vi "Create Hardware Configuration.vi"   [LabVIEW 2018]
uses:
  Resources/Type Defs/Stage Configuration.ctl
  Resources/Type Defs/Microscope Configuration.ctl
  Resources/Type Defs/Microscope Type.ctl
  Resources/Type Defs/Virtual Camera Configuration.ctl
  Resources/Type Defs/Camera Type.ctl
  Resources/Type Defs/Laser Configuration.ctl
  Resources/Type Defs/Pump Configuration.ctl
  Resources/Type Defs/Hardware Configuration.ctl
  Resources/Type Defs/Shutter Configuration.ctl
  Resources/Type Defs/Physical Camera Assignment.ctl
  <vilib>/Utility/xml.llb/Write to XML File(string).vi
panel:
  # "Open the Block Diagram (Ctrl-E)\nto edit configuration settings."
types:
  T1 = typedef "Shutter Configuration.ctl" = cluster{"IO Line":tag, "Name":string, "Wavelength":u16, "Max rate (Hz)":dbl}
  T2 = typedef "Physical Camera Assignment.ctl" = cluster{"Channel Name":string, "Camera Type":T3, "Serial Number":string, "Flip Vertically":bool, "Flip Horizontally":bool, "photonsPerCount":dbl, "wavelength":i16}
  T3 = typedef "Camera Type.ctl" = enum16{"Hamamatsu"}
  T4 = typedef "Hardware Configuration.ctl" = cluster{"Shutters":T1[], "Stage Configuration":T5, "Microscope Configuration":T6, "Virtual Camera Configuration":T8, "Laser Configuration":T9[], "Fluidics Configuration":T10, "Installed Cameras":T2[]}
  T5 = typedef "Stage Configuration.ctl" = cluster{"Serial Port":refnum<visa-resource-name>, "Forward Step (mm)":dbl, "Lane Length (mm)":dbl, "Lane Separation (mm)":dbl, "Stage Type":enum16{"Disabled", "ESP301", "Ti2"}}
  T6 = typedef "Microscope Configuration.ctl" = cluster{"Serial Port":refnum<visa-resource-name>, "Microscope Type":T7, "Detection Settings":cluster{"Name":string, "Filter Position":u16, "Optical Path":u16}[]}
  T7 = typedef "Microscope Type.ctl" = enum16{"Disable", "TE2000", "Eclipse Ti", "Ti2"}
  T8 = typedef "Virtual Camera Configuration.ctl" = cluster{"Camera Type":T3, "Sync Line":tag}
  T9 = typedef "Laser Configuration.ctl" = cluster{"Serial Port":refnum<visa-resource-name>, "Laser Type":enum16{"Disable", "Laser Quantum", "Coherent OBIS", "PRM1-Z8"}, "Polarizer Amplitude":dbl, "Polarizer Theta Zero":dbl, "Wavelength":u16}
  T10 = typedef "Pump Configuration.ctl" = cluster{"Fluidics present":bool}
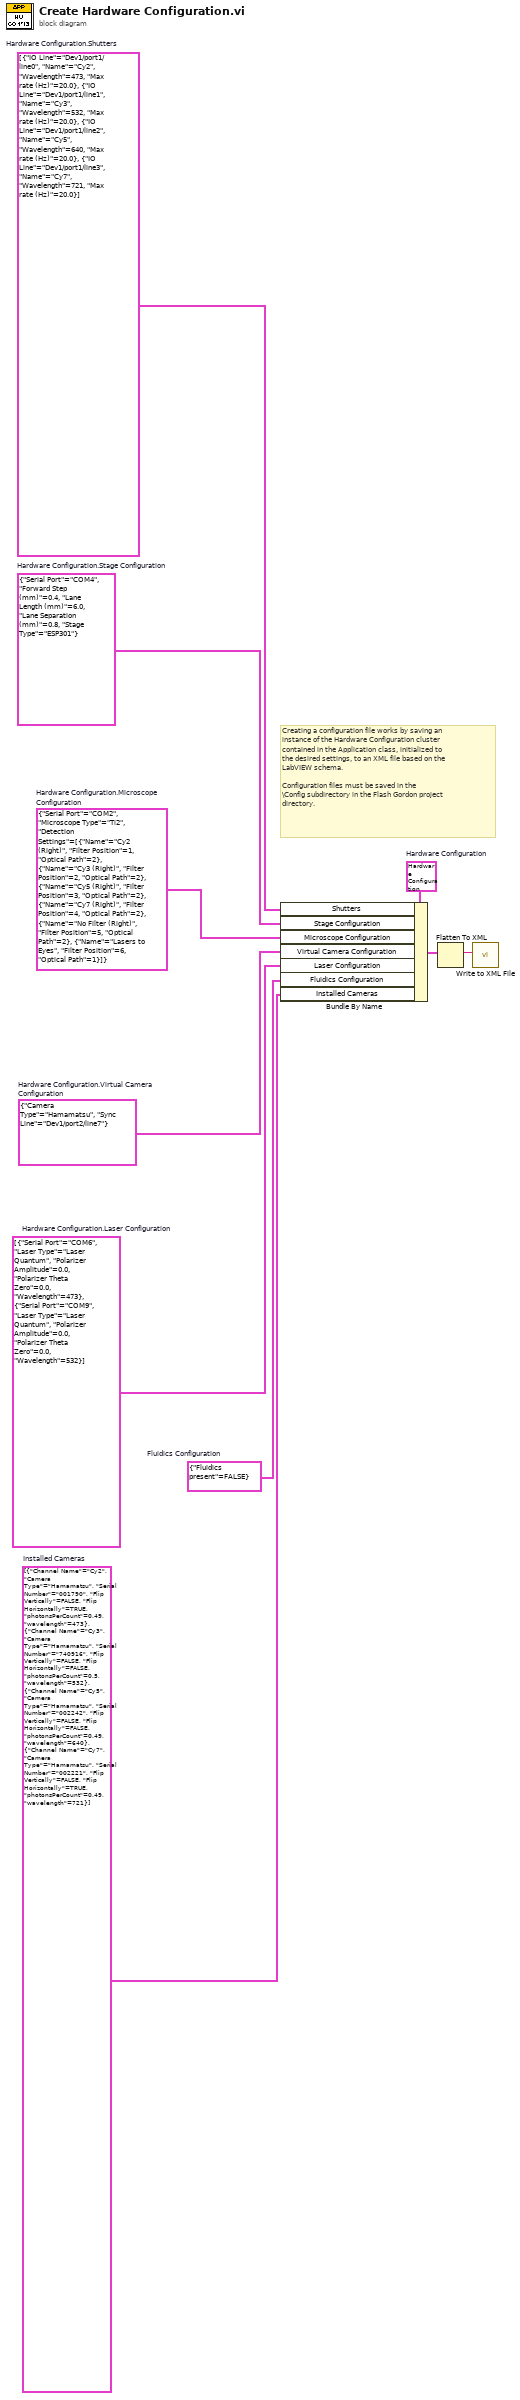
[diagram p0: block diagram]
diagram:
  w1 = T1[] [{"IO Line"="Dev1/port1/line0", "Name"="Cy2", "Wavelength"=473, "Max rate (Hz)"=20.0}, {"IO Line"="Dev1/port1/line1", "Name"="Cy3", "Wavelength"=532, "Max rate (Hz)"=20.0}, {"IO Line"="Dev1/port1/line2", "Name"="Cy5", "Wavelength"=640, "Max rate (Hz)"=20.0}, {"IO Line"="Dev1/port1/line3", "Name"="Cy7", "Wavelength"=721, "Max rate (Hz)"=20.0}]  # Hardware Configuration.Shutters
  w2 = T2[] [{"Channel Name"="Cy2", "Camera Type"=enum."Hamamatsu", "Serial Number"="001790", "Flip Vertically"=FALSE, "Flip Horizontally"=TRUE, "photonsPerCount"=0.49, "wavelength"=473}, {"Channel Name"="Cy3", "Camera Type"=enum."Hamamatsu", "Serial Number"="740916", "Flip Vertically"=FALSE, "Flip Horizontally"=FALSE, "photonsPerCount"=0.5, "wavelength"=532}, {"Channel Name"="Cy5", "Camera Type"=enum."Hamamatsu", "Serial Number"="002242", "Flip Vertically"=FALSE, "Flip Horizontally"=FALSE, "photonsPerCount"=0.49, "wavelength"=640}, {"Channel Name"="Cy7", "Camera Type"=enum."Hamamatsu", "Serial Number"="002221", "Flip Vertically"=FALSE, "Flip Horizontally"=TRUE, "photonsPerCount"=0.49, "wavelength"=721}]  # Installed Cameras
  w3 = T4 {"Shutters"=[], "Stage Configuration"={"Serial Port"="COM3", "Forward Step (mm)"=0.4, "Lane Length (mm)"=6.0, "Lane Separation (mm)"=0.8, "Stage Type"=enum."ESP301"}, "Microscope Configuration"={"Serial Port"="COM2", "Microscope Type"=enum."TE2000", "Detection Settings"=[]}, "Virtual Camera Configuration"={"Camera Type"=enum."Hamamatsu", "Sync Line"=""}, "Laser Configuration"=[], "Fluidics Configuration"={"Fluidics present"=FALSE}, "Installed Cameras"=[]}  # Hardware Configuration
  w4 = T10 {"Fluidics present"=FALSE}  # Fluidics Configuration
  w6 = T9[] [{"Serial Port"="COM6", "Laser Type"=enum."Laser Quantum", "Polarizer Amplitude"=0.0, "Polarizer Theta Zero"=0.0, "Wavelength"=473}, {"Serial Port"="COM9", "Laser Type"=enum."Laser Quantum", "Polarizer Amplitude"=0.0, "Polarizer Theta Zero"=0.0, "Wavelength"=532}]  # Hardware Configuration.Laser Configuration
  w7 = T8 {"Camera Type"=enum."Hamamatsu", "Sync Line"="Dev1/port2/line7"}  # Hardware Configuration.Virtual Camera Configuration
  w8 = T6 {"Serial Port"="COM2", "Microscope Type"=enum."Ti2", "Detection Settings"=[{"Name"="Cy2 (Right)", "Filter Position"=1, "Optical Path"=2}, {"Name"="Cy3 (Right)", "Filter Position"=2, "Optical Path"=2}, {"Name"="Cy5 (Right)", "Filter Position"=3, "Optical Path"=2}, {"Name"="Cy7 (Right)", "Filter Position"=4, "Optical Path"=2}, {"Name"="No Filter (Right)", "Filter Position"=5, "Optical Path"=2}, {"Name"="Lasers to Eyes", "Filter Position"=6, "Optical Path"=1}]}  # Hardware Configuration.Microscope Configuration
  w9 = T5 {"Serial Port"="COM4", "Forward Step (mm)"=0.4, "Lane Length (mm)"=6.0, "Lane Separation (mm)"=0.8, "Stage Type"=enum."ESP301"}  # Hardware Configuration.Stage Configuration
  # "Creating a configuration file works by saving an\ninstance of the Hardware Configuration cluster\ncontained in the Application class, initialized to \nthe desired settings, to an XML file based on the \nLabVIEW schema.\n\nConfiguration files must be saved in the\n\\Config subdirectory in the Flash Gordon project\ndirectory."
  n1 = Bundle By Name(cluster=w3, "Shutters"=w1, "Stage Configuration"=w9, "Microscope Configuration"=w8, "Virtual Camera Configuration"=w7, "Laser Configuration"=w6, "Fluidics Configuration"=w4, "Installed Cameras"=w2) -> (w10:T4)
  n2 = Flatten To XML(anything=w10) -> (xml string=w5:string)
  n3 = call-poly <vilib>:"Write to XML File.vi"("XML Input"=w5) -> ()  [unwired: 8 in, 3 out]
